vi "Configure.vi"(8 "error in (no error)":errorcluster, 11 "Device in":refnum<class "Device.lvclass">) -> (0 "error out":errorcluster, 3 "Device out":refnum<class "Device.lvclass">)   [LabVIEW 2020, in "Device.lvlib" / "Device.lvclass"]
uses:
  Device.lvclass
  GenericActor/GenericActor/GenericActor.lvclass
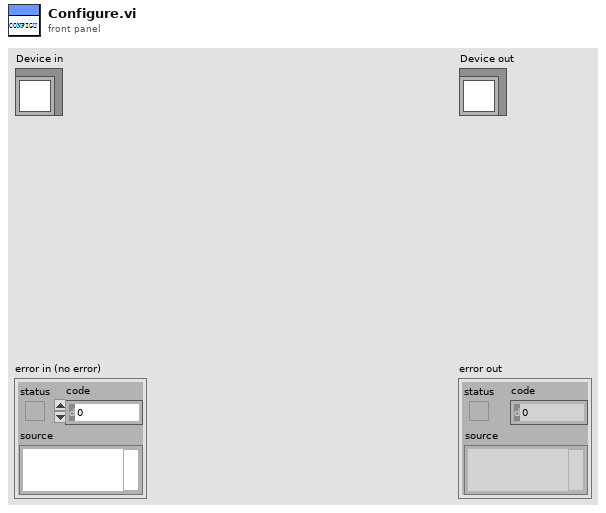
[diagram p1: front panel]
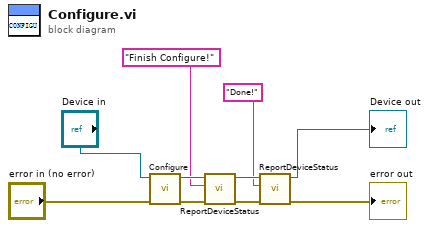
[diagram p0: block diagram]
diagram:
  n1 = call-parent "Configure.vi"("error in (no error)"="error in (no error)", "GRMActor in"="Device in") -> ("error out"=w10:errorcluster, "GRMActor out"=w4:refnum<class "Device.lvclass">)  [unwired: 8 in]
  n2 = call-dynamic "ReportDeviceStatus.vi"("error in (no error)"=w10, "Status"="Finish Configure!", "Device in"=w4) -> ("error out"=w5:errorcluster, "Device out"=w3:refnum<class "Device.lvclass">)  [unwired: 7 in]
  n3 = call-dynamic "ReportDeviceStatus.vi"("error in (no error)"=w5, "Status"="Done!", "Device in"=w3) -> ("error out"=→"error out":errorcluster, "Device out"=→"Device out":refnum<class "Device.lvclass">)  [unwired: 7 in]
